vi "convert_sched_to_legacy.vi"(10 "Team Info":T1, 11 "Match Array (indices)":i32[][](array[numeric])) -> ()   [LabVIEW 2013]
uses:
  Team Data Array.ctl
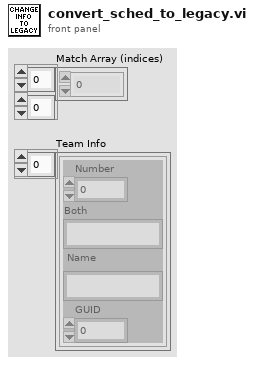
[diagram p1: front panel]
types:
  T1 = typedef "Team Data Array.ctl" = cluster{"Number":u16, "Both":string, "Name":string, "GUID":u16}[]
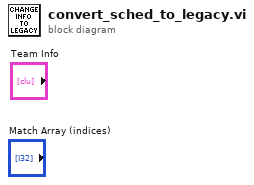
[diagram p0: block diagram]
diagram:
